vi "PS_Signal_Gen_Command.vi"(10 "Value String":string, 11 "Command String":string) -> (0 "error out":errorcluster, 2 "Read Back":string, 3 "Request String":string)   [LabVIEW 2011]
uses:
  PS_Global.vi
  <vilib>/Instr/_visa.llb/VISA Configure Serial Port (Instr).vi
panel:
  in  "baud rate":u32=115200
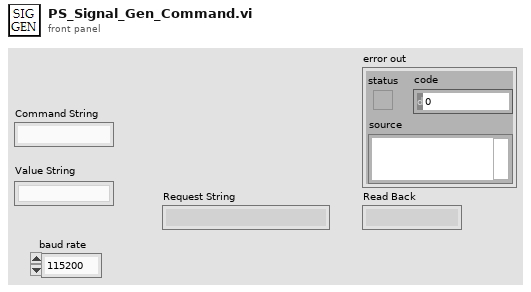
[diagram p1: front panel]
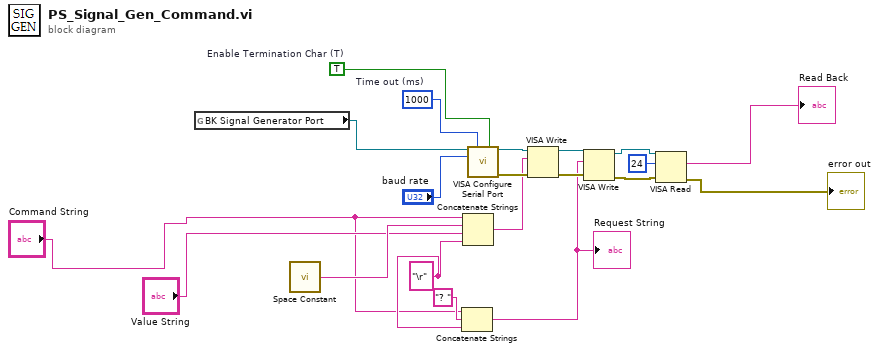
[diagram p0: block diagram]
diagram:
  w2 = "\r"
  w16 = TRUE  # Enable Termination Char (T)
  w19 = 1000  # Time out (ms)
  n1 = global read "PS_Global.vi" "BK Signal Generator Port"() -> (w14:refnum<visa-resource-name>)
  n2 = call <vilib>:"Space Constant.vi"() -> ("String"=w13:string)
  n3 = Concatenate Strings("Command String", "? " ("string"), w2) -> (w8:string)
  "Request String" <- w8
  n4 = Concatenate Strings("Command String", w13, "Value String", w2) -> (w15:string)
  n5 = call-poly "VISA Configure Serial Port"("VISA resource name"=w14, "timeout (10sec)"=w19, "Enable Termination\nChar (T)"=w16, "baud rate (9600)"="baud rate") -> ("VISA resource name out"=w18:refnum<visa-resource-name>, "error out"=w17:errorcluster)  [unwired: 10 in]
  n6 = VISA Write(VISA resource name=w18, write buffer=w15, error in (no error)=w17) -> (VISA resource name out=w11:refnum<visa-resource-name>, error out=w12:errorcluster)  [unwired: 1 out]
  n7 = VISA Write(VISA resource name=w11, write buffer=w8, error in (no error)=w12) -> (VISA resource name out=w6:refnum<visa-resource-name>, error out=w5:errorcluster)  [unwired: 1 out]
  n8 = VISA Read(VISA resource name=w6, byte count=u32 24, error in (no error)=w5) -> (read buffer=→"Read Back":string, error out=→"error out":errorcluster)  [unwired: 2 out]
